vi "Simple.vi"() -> ()   [LabVIEW 2012]
panel:
  out "Altitude 3":dbl=88890.0
  in  "Confirm Now":bool
  in  "RUN":bool=TRUE
  in  "Altitude 2":dbl=88890.0
  out "Altitude":dbl=88888.0
  in  "Cluster":T1
  # "Project and room name"
  # "F\ne\ne\nt"
  # "%"
  # "HOLD"
  # "CO2"
  # "OFF"
  # "Set-up"
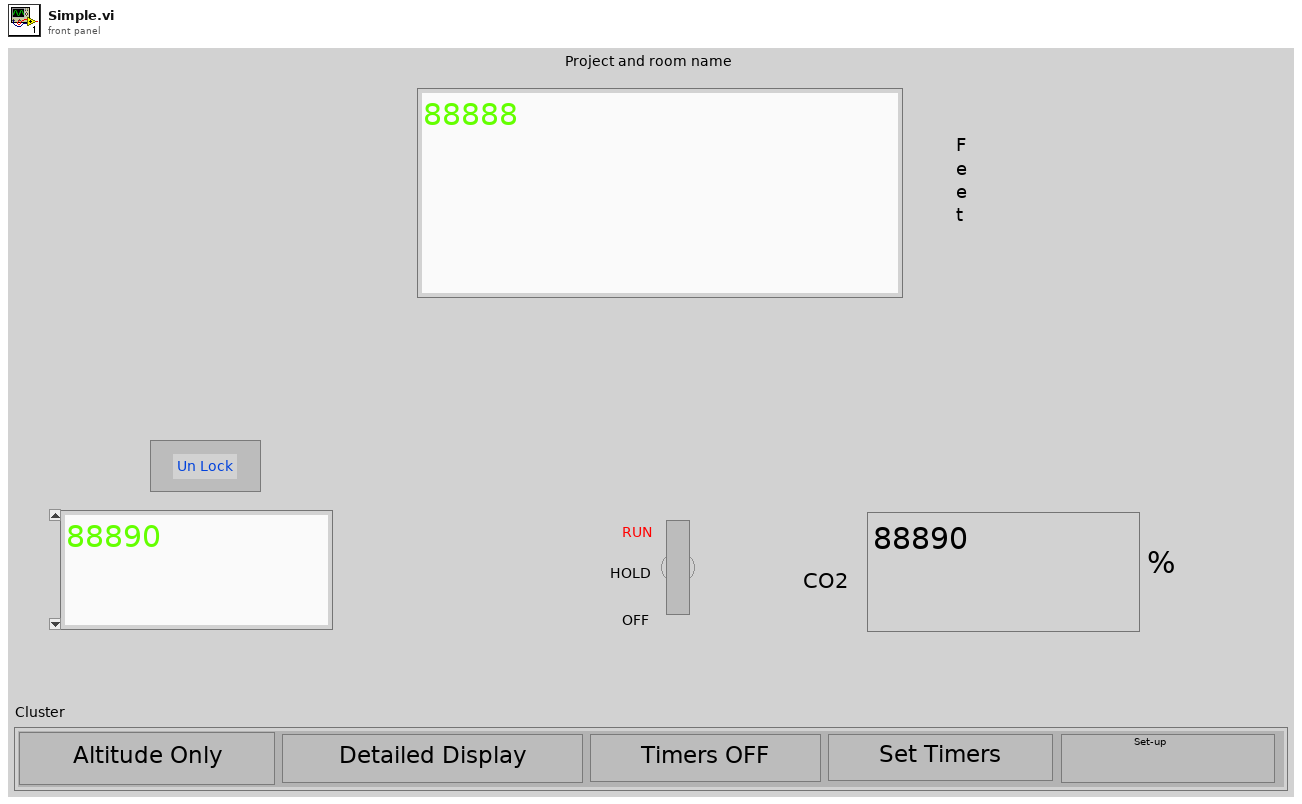
[diagram p1: front panel]
types:
  T1 = cluster{"OK Button":bool, "OK Button 2":bool, "OK Button":bool, "OK Button 4":bool, "OK Button 3":bool}
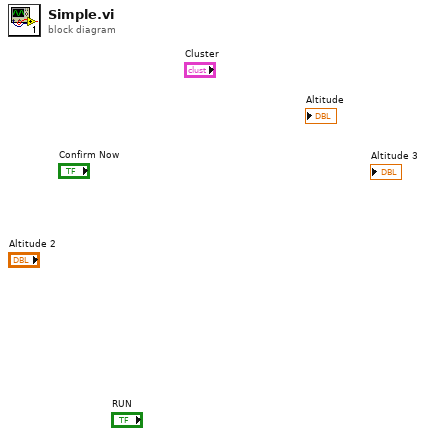
[diagram p0: block diagram]
diagram:
